vi "Initialize.vi"(7 "Limit Name":string="Setpoint.ch%d.SP", 8 "error in":errorcluster, 9 "Number of Channels":u32=1, 10 "Instance Name":string="PluginName", 11 "Pressure Limit in":refnum<class "Pressure Limit.lvclass">) -> (0 "error out":errorcluster caption="error in", 3 "Pressure Limit out":refnum<class "Pressure Limit.lvclass">)   [LabVIEW 2023, in "Pressure Limit.lvclass"]
uses:
  Pressure Limit.lvclass
  Pressure Limit.lvclass/Pressure Limit.ctl
  Parents/Limit/Limit.lvclass
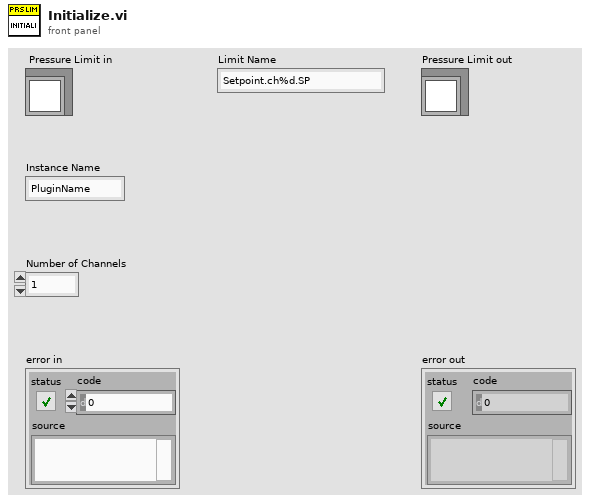
[diagram p1: front panel]
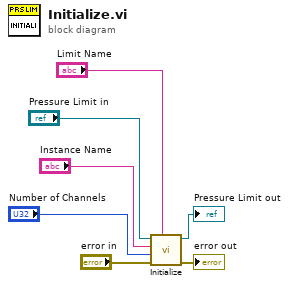
[diagram p0: block diagram]
diagram:
  n1 = call-parent "Initialize.vi"("Limit Name"="Limit Name", "error in"="error in", "Number of Channels"="Number of Channels", "Instance Name"="Instance Name", "Limit in"="Pressure Limit in") -> ("error out"=→"error out":errorcluster, "Limit out"=→"Pressure Limit out":refnum<class "Pressure Limit.lvclass">)  [unwired: 5 in]
